vi "Get Random Number.vi"(8 "error in (no error)":errorcluster, 11 "Worker in":refnum<class "Worker.lvclass">) -> (0 "error out":errorcluster, 3 "Worker out":refnum<class "Worker.lvclass">)   [LabVIEW 2024, in "Worker.lvlib" / "Worker.lvclass"]
uses:
  Worker.lvclass
  Worker.lvclass/Worker.ctl
  <vilib>/numeric/Random Number (Range) U64.vi
  <vilib>/ActorFramework/Actor/Actor.lvclass
  Chef State Logic/Work Logic Messages/Update Count Msg/Update Count Msg.lvclass
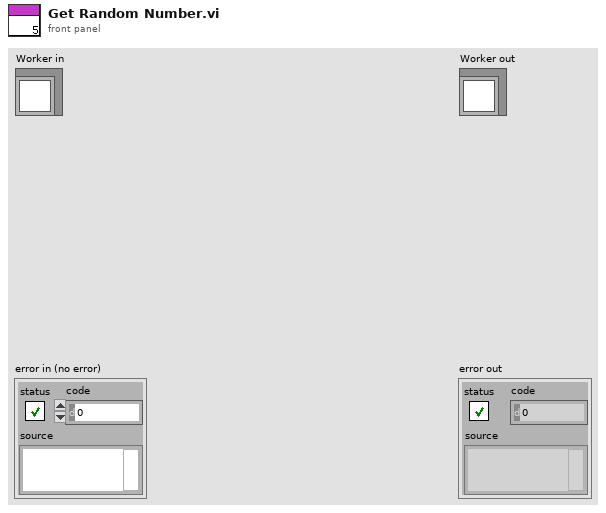
[diagram p1: front panel]
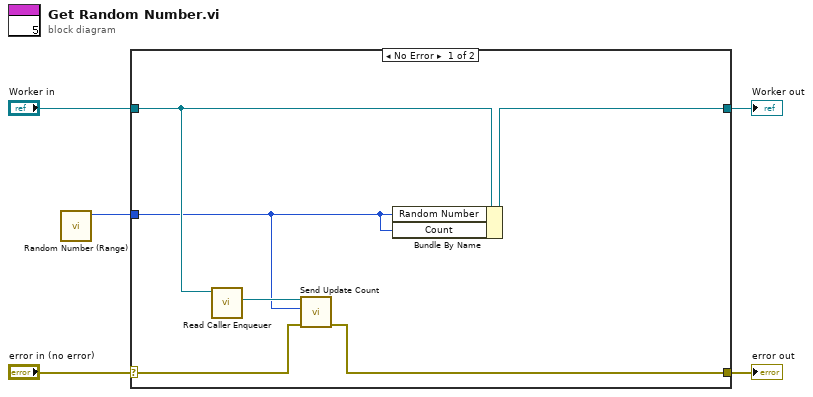
[diagram p0: block diagram]
diagram:
  n1 = call-poly <vilib>:"Random Number (Range).vi"() -> ("number"=w1:u64)  [unwired: 11 in]
  n2 = case shown="No Error" "error in (no error)" {
    selector: "error in (no error)" -> [w9 w13]
    tunnel: [w8 w13] -> w4
    tunnel: [w11 w12] -> w2
    tunnel: "Worker in" -> [w10 w12]
    tunnel: w1 -> [w6 _]
    frame No Error {
      n3 = call <vilib>:"Read Caller Enqueuer.vi"("Actor"=w10) -> ("Caller Enqueuer"=w7:refnum<class "Message Enqueuer.lvclass">)  [unwired: 10 in]
      n4 = call "Send Update Count.vi"("error in (no error)"=w9, "Numeric"=w6, "Message Enqueuer"=w7) -> ("error out"=w8:errorcluster)  [unwired: 7 in, 1 out]
      n5 = Bundle By Name(cluster=w10, "Random Number"=w6, "Count"=w6) -> (w11:refnum<class "Worker.lvclass">)
    }
    frame Error {
    }
  }
  "error out" <- w4
  "Worker out" <- w2
